vi "Manual Test.vi"() -> ()   [LabVIEW 2023]
panel:
  in  "String":string="{ \"hello\":\"world\", \"test\":\"bananas\",\"number\":554}"
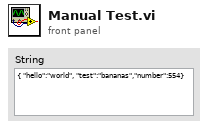
[diagram p1: front panel]
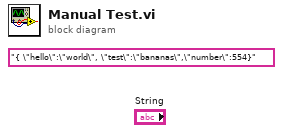
[diagram p0: block diagram]
diagram:
  (unwired) "{ \"hello\":\"world\", \"test\":\"bananas\",\"number\":554}"
